vi "Read data member B.vi"(8 "error in (no error)":errorcluster, 11 "Sample Class in":refnum<class "Sample Class.lvclass">) -> (0 "error out":errorcluster, 2 "data member B":string, 3 "Sample Class out":refnum<class "Sample Class.lvclass">)   [LabVIEW 2023, in "Sample Class.lvclass"]
doc: "Reads the value of Data member B in an instance of Sample Class."
uses:
  Sample Class.lvclass
  Sample Class.lvclass/Sample Class.ctl
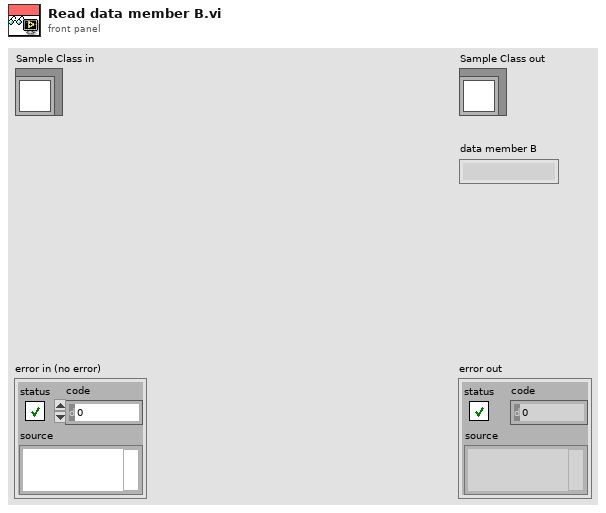
[diagram p1: front panel]
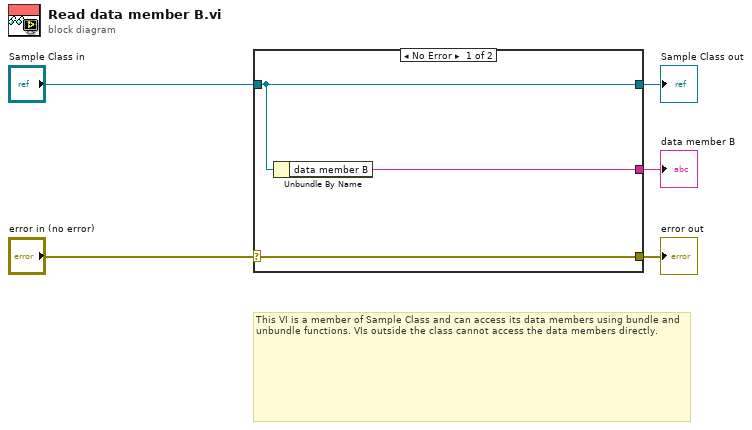
[diagram p0: block diagram]
diagram:
  # "This VI is a member of Sample Class and can access its data members using bundle and unbundle functions. VIs outside the class cannot access the data members directly."
  n1 = case shown="No Error" "error in (no error)" {
    selector: "error in (no error)" -> [w8 w9]
    tunnel: [w8 w9] -> w4
    tunnel: [w7 w10] -> w2
    tunnel: "Sample Class in" -> [w7 w10]
    tunnel: [w6 _] -> w1
    frame No Error {
      n2 = Unbundle By Name(w7) -> ("data member B"=w6:string)
    }
    frame Error {
    }
  }
  "error out" <- w4
  "Sample Class out" <- w2
  "data member B" <- w1
